vi "Step Simulation.vi"(0 "reference in":refnum<class "Battery.lvclass">, 1 "current_A":dbl=1.0, 2 "time_step_S":dbl=0.0015 format="%#_13g", 5 "Error In":errorcluster) -> (14 "reference out":refnum<class "Battery.lvclass">, 15 "open circuit voltage":dbl, 16 "state of charge":dbl, 19 "Error Out":errorcluster)   [LabVIEW 2023, in "Battery.lvclass"]
uses:
  Battery.lvclass
  Battery.lvclass/Battery.ctl
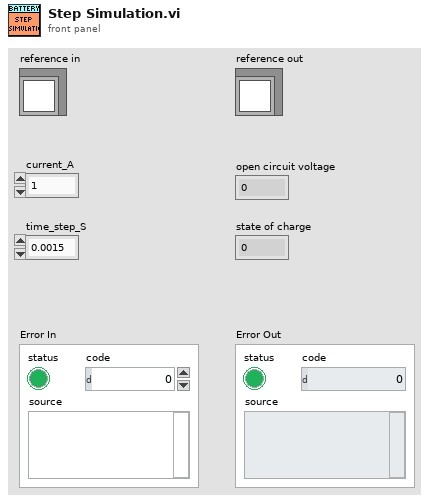
[diagram p1: front panel]
types:
  T1 = typedef "Battery.lvclass/ObjectAttributes.ctl" = cluster{"Python module":path, "Python Session":refnum<k35>, "PybammWrapper":refnum<k38>, "model loaded":bool, "simulation loaded":bool, "simulation enabled":bool, "SOC OCV Curve":dbl[][], "Open Circuit Voltage (V)":dbl, "State of Charge (%)":dbl, "# Cells in Series":u16, "# Cells in Parallel":u16, "Model Parameters":T2, "Simulation Parameters":T3, "Power Module":refnum<class "PowerModuleInterface.lvclass">}
  T2 = typedef "Battery.lvclass/Model Parameters.ctl" = cluster{"chemistry":string, "model_type":string}
  T3 = typedef "Battery.lvclass/Simulation Parameters.ctl" = cluster{"num_rc_pairs":i32, "R0":dbl, "R1":dbl, "C1":dbl, "R2":dbl, "C2":dbl, " nominal_capacity_Ah":dbl, "upper_voltage_cutoff":dbl, "lower_voltage_cutoff":dbl}
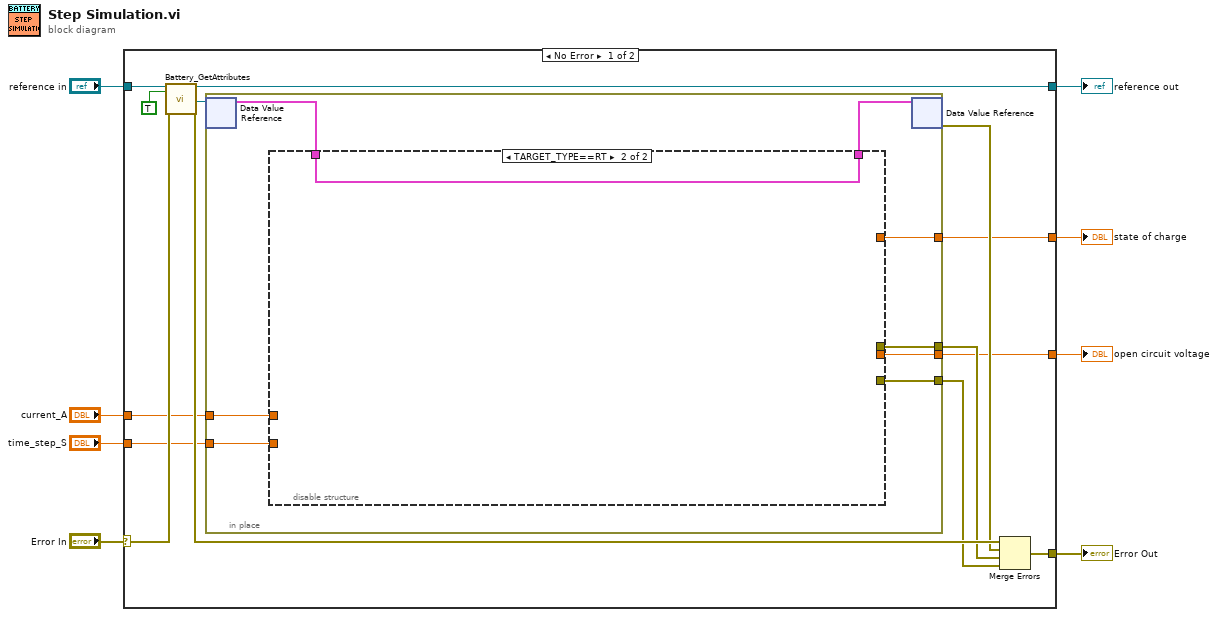
[diagram p0: block diagram]
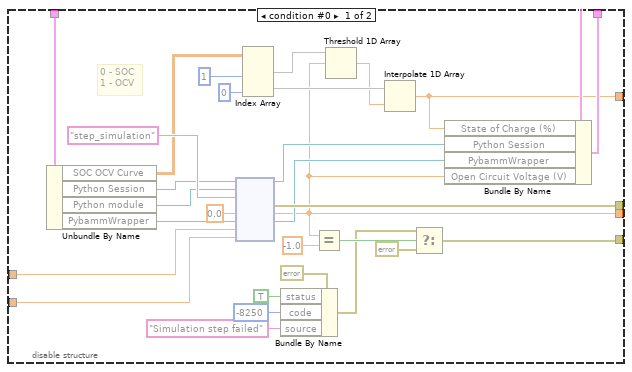
[diagram p2: hidden frame]
diagram:
  n1 = case shown="No Error" "Error In" {
    selector: "Error In" -> [w21 w62]
    tunnel: [w19 w62] -> w7
    tunnel: [w20 w61] -> w5
    tunnel: "reference in" -> [w22 w61]
    tunnel: [w13 _] -> w4
    tunnel: "current_A" -> [w12 _]
    tunnel: "time_step_S" -> [w11 _]
    tunnel: [w10 _] -> w1
    frame No Error {
      n2 = call "Battery_GetAttributes.vi"("reference in"=w22, "OnlyGetDvrReference(False)"=TRUE, "Error In"=w21) -> ("reference out"=w20:refnum<class "Battery.lvclass">, "DataRef"=w18:refnum<data-value>, "Error Out"=w16:errorcluster)  [unwired: 13 in, 1 out]
      n3 = in-place {
        in-place-border: [w30] -> w14
        in-place-border: [w24] -> w13
        in-place-border: w12 -> [w27]
        in-place-border: w11 -> [w26]
        in-place-border: [w25] -> w10
        in-place-border: [w23] -> w9
        n4 = in-place-dvr #1(w18) -> (w29:T1)  [unwired: 1 out]
        n5 = disable-structure shown="TARGET_TYPE==RT" {
          disable-tunnel: [w58 _] -> w30
          disable-tunnel: w29 -> [w54 w60]
          disable-tunnel: [w51 w60] -> w28
          disable-tunnel: w27 -> [w50 _]
          disable-tunnel: w26 -> [w48 _]
          disable-tunnel: [w43 _] -> w25
          disable-tunnel: [w40 _] -> w24
          disable-tunnel: [w31 _] -> w23
          frame condition #0 {
            # "0 - SOC\n1 - OCV"
            n6 = Unbundle By Name(w54) -> ("SOC OCV Curve"=w47:dbl[][], "Python Session"=w55:refnum<k35>, "Python module"=w56:path, "PybammWrapper"=w57:refnum<k38>)
            n7 = node(w55, w56, "step_simulation" ("function name"), 0.0 ("current_A"), w57, w50, w48) -> (w53:refnum<k35>, w58:errorcluster, w40:dbl, w52:refnum<k38>)  [unwired: 3 in, 2 out]
            n8 = Index Array(array=w47, index (col) #1=1 ("disabled index (col)"), index (col) #2=0 ("disabled index (col)")) -> (element #1=w45:dbl[], element #2=w46:dbl[])  [unwired: 2 in]
            n9 = Bundle By Name(cluster=errorcluster {"status"=FALSE, "code"=0, "source"=""} ("error out"), "status"=TRUE, "code"=-8250, "source"="Simulation step failed") -> (w33:errorcluster)
            n10 = Equal?(x=w40, y=-1.0) -> (x = y?=w34:bool)
            n11 = Threshold 1D Array(2:w40, 3:w45) -> (0:w44:dbl)  [unwired: 1 in]
            n12 = Interpolate 1D Array(1:w44, 2:w46) -> (0:w43:dbl)
            n13 = Select(t=w33, s=w34, f=errorcluster {"status"=FALSE, "code"=0, "source"=""}) -> (s? t:f=w31:errorcluster)
            n14 = Bundle By Name(cluster=w54, "State of Charge (%)"=w43, "Python Session"=w53, "PybammWrapper"=w52, "Open Circuit Voltage (V)"=w40) -> (w51:T1)
          }
          frame condition #1 (active) {
          }
        }
        n15 = in-place-dvr #1(w28) -> (w15:errorcluster)  [unwired: 1 out]
      }
      n16 = Merge Errors(w16, w15, w14, w9) -> (w19:errorcluster)
    }
    frame Error {
    }
  }
  "Error Out" <- w7
  "reference out" <- w5
  "open circuit voltage" <- w4
  "state of charge" <- w1
